vi "AIClient.vi"() -> ()   [LabVIEW 2025]
uses:
  AIGlobalqueue.vi
panel:
  in  "get_action":bool
  out "ACTION":T1
  in  "reset":bool
  out "Numeric 2":i32
  in  "stop":bool
  in  "updateforward":bool
  out "action name":string
  in  "action":i32
  in  "map_size":i32
  out "reset_agent output":i32
  out "action":i32
  out "y":i32
  out "x":i32
  in  "Array 2":i32[](array[numeric])
  out "Array":i32[](array[numeric])
  in  "player_ID":i32
  in  "armies_map":i32[][](array[numeric])
  in  "owner_map":i32[][](array[numeric])
  out "initialize output":i32
  out "error out":errorcluster
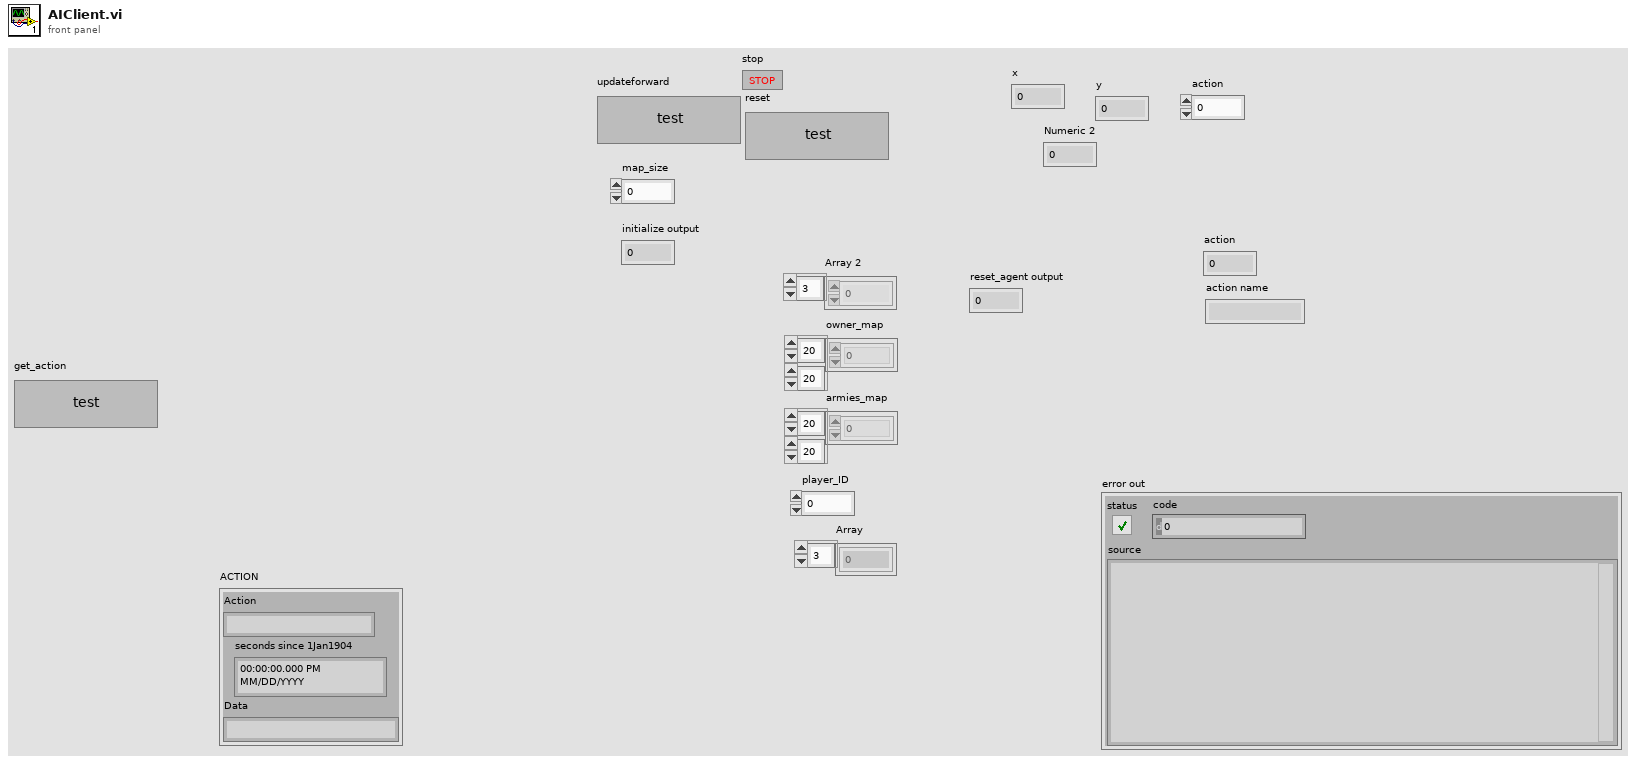
[diagram p1: front panel]
types:
  T1 = cluster{"Action":string, "seconds since 1Jan1904":timestamp, "Data":string}
  T2 = cluster{"seconds since 1Jan1904":timestamp, "Data":string}
  T3 = cluster{"owner_map":i32[][], "armies_map":i32[][], "turn_ID":i32, "player_ID":i32}
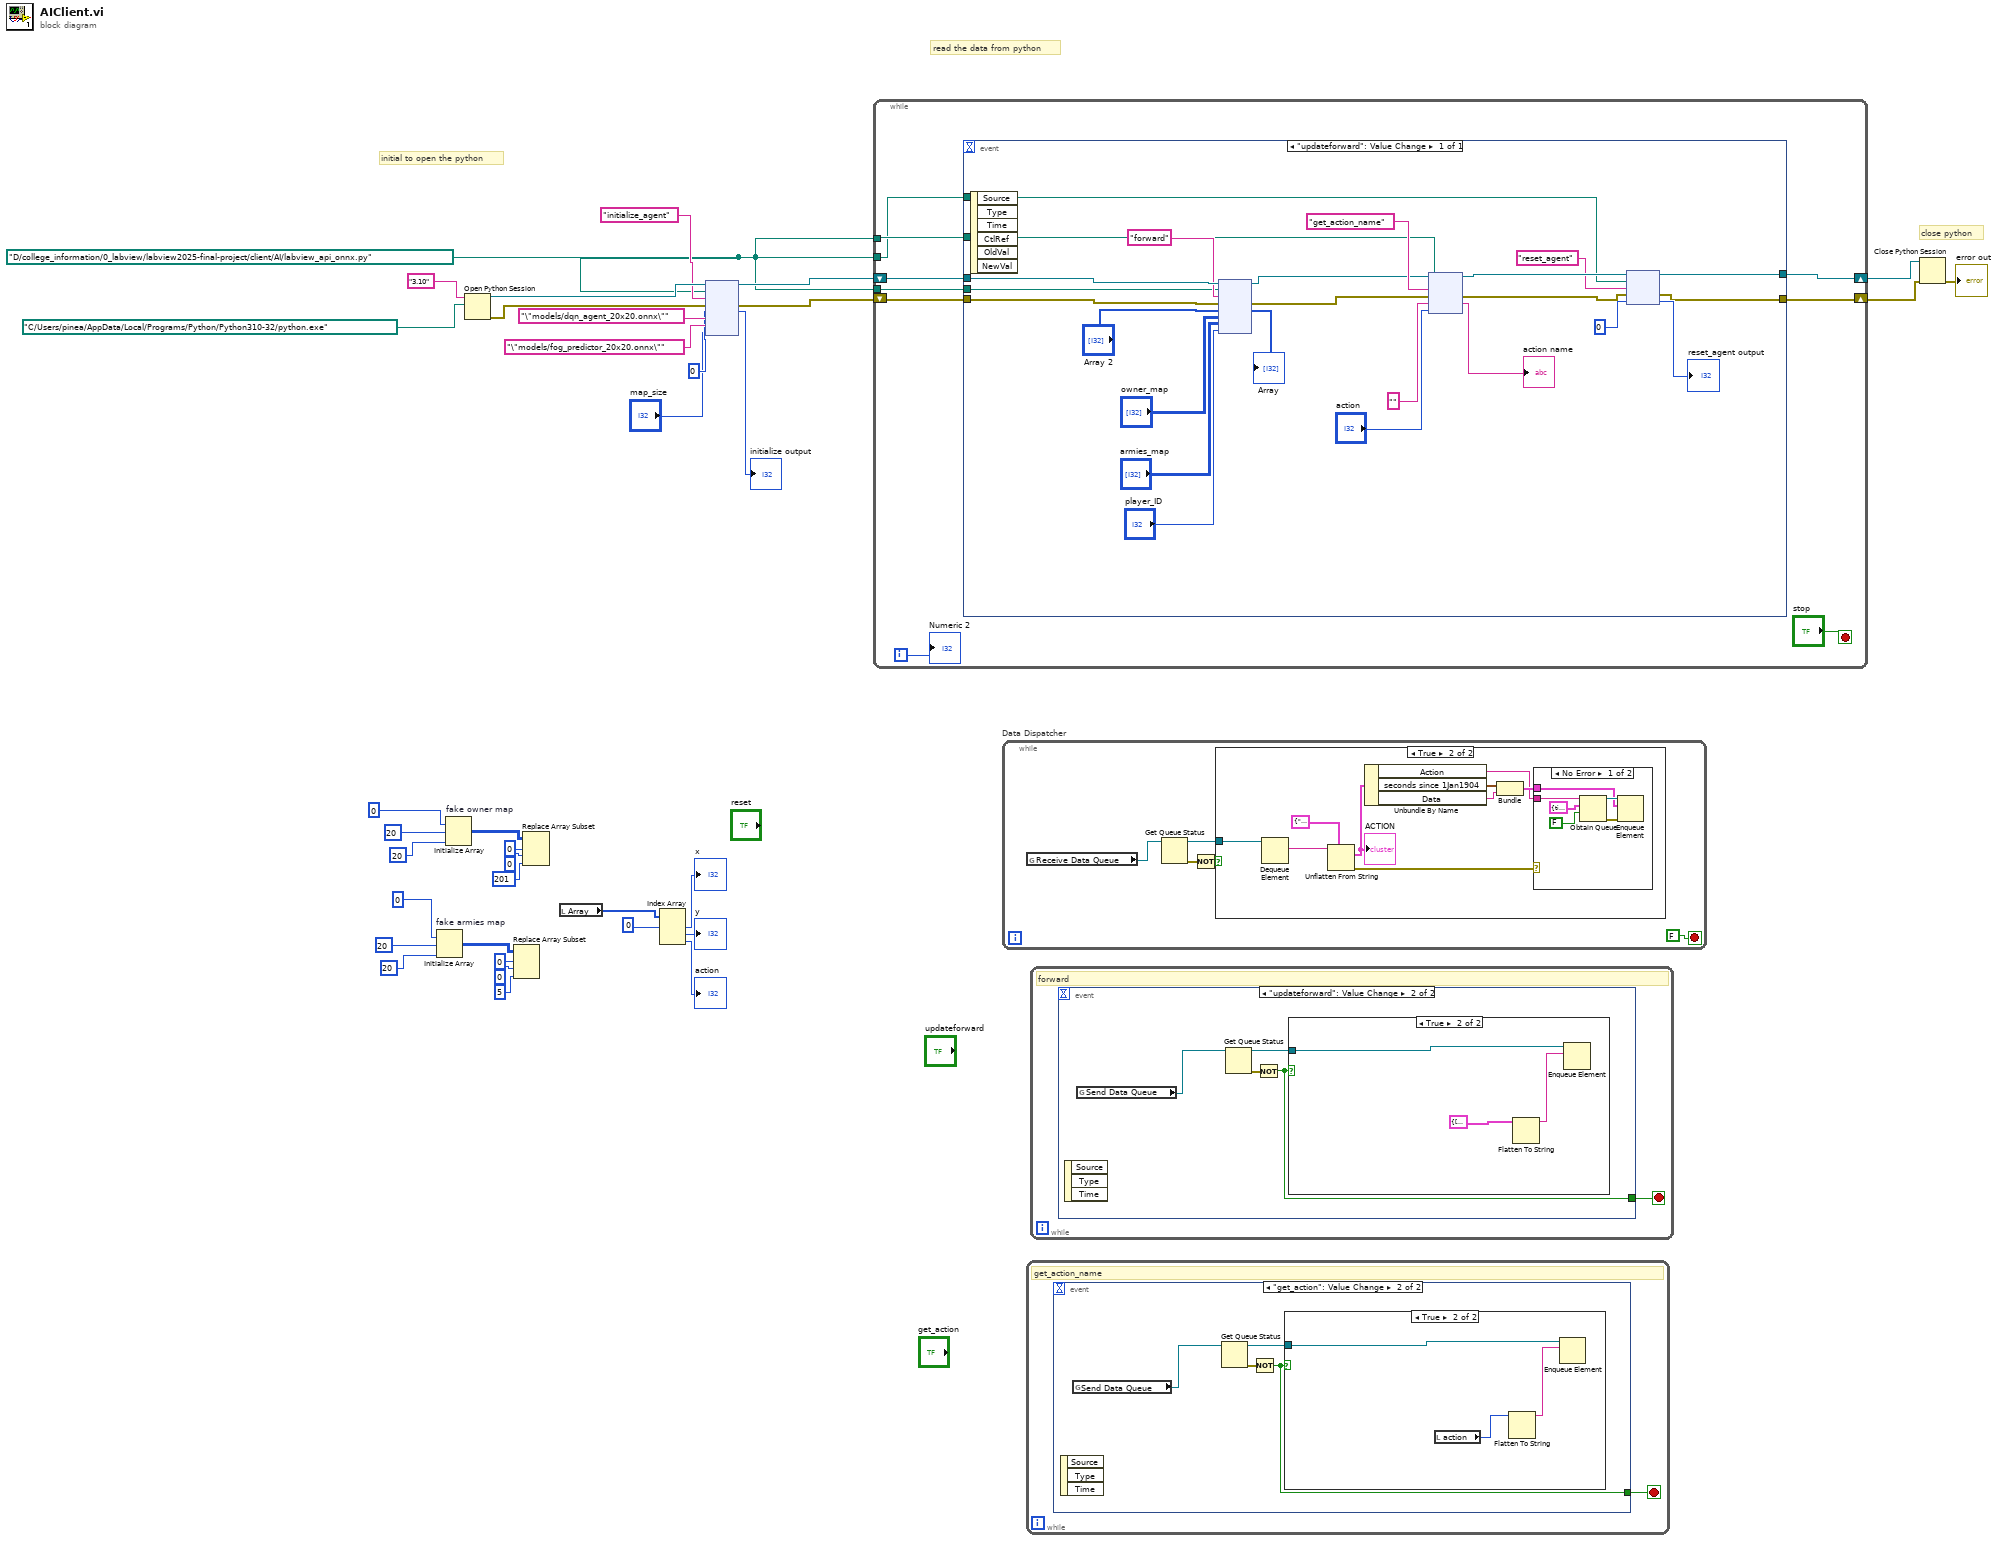
[diagram p0: block diagram]
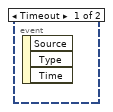
[diagram p2: hidden frame]
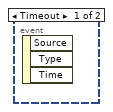
[diagram p4: hidden frame]
diagram:
  w17 = path "D:/college_information/0_labview/labview2025-final-project/client/AI/labview_api_onnx.py" ("Python path")
  # "read the data from python"
  # "close python"
  # "initial to open the python"
  n1 = Initialize Array "fake armies map"(0 ("element"), 20 ("dimension size"), 20 ("dimension size")) -> (w14:i32[][])
  n2 = Initialize Array "fake owner map"(0 ("element"), 20 ("dimension size"), 20 ("dimension size")) -> (w13:i32[][])
  n3 = Open Python Session(python version="3.10" ("Python version"), python path=path "C:/Users/pinea/AppData/Local/Programs/Python/Python310-32/python.exe" ("Python path")) -> (session out=w34:refnum<k35>, error out=w33:errorcluster)  [unwired: 1 in]
  n4 = Replace Array Subset(array=w14, new element=5 ("new element/subarray"), index (row)=0, index (col)=0 ("disabled index (col)")) -> ()  [unwired: 1 out]
  n5 = Replace Array Subset(array=w13, new element=201 ("new element/subarray"), index (row)=0, index (col)=0 ("disabled index (col)")) -> ()  [unwired: 1 out]
  n6 = local read "Array"() -> (w30:i32[])
  n7 = Index Array(array=w30, index #1=0 ("index")) -> (element #1=→"x":i32, element #2=→"y":i32, element #3=→"action":i32)  [unwired: 2 in]
  n8 = node(w34, w17, "initialize_agent" ("function name"), w33, 0, "\"models/dqn_agent_20x20.onnx\"", "\"models/fog_predictor_20x20.onnx\"", "map_size") -> (w20:refnum<k35>, w19:errorcluster, →"initialize output":i32)  [unwired: 3 in, 2 out]
  n9 = while {
    tunnel: w17 -> [w42]
    shift-right: [w37] -> w16
    shift-left: w20 -> [w44]
    shift-right: [w36] -> w15
    shift-left: w19 -> [w43]
    tunnel: w17 -> [w41]
    tunnel: w17 -> [w38]
    i -> [w39]
    stop <- "stop" stop-if-true
    n10 = event shown="[0] \"updateforward\": Value Change" {
      selector: _ -> [_]
      dyn-events: _ -> [_]
      timeout: _ -> [_]
      tunnel: w44 -> [w64]
      tunnel: w43 -> [w63]
      tunnel: w42 -> [w57]
      tunnel: w41 -> [w56]
      tunnel: w38 -> [w53]
      tunnel: [w49] -> w37
      tunnel: [w48] -> w36
      event "updateforward": Value Change {
        n11 = event-data() -> ()  [unwired: 1 in, 6 out]
        n12 = node(w64, w57, "forward" ("function name"), w63, "Array 2", "owner_map", "armies_map", "player_ID") -> (w59:refnum<k35>, w58:errorcluster, →"Array":i32[])  [unwired: 3 in, 2 out]
        n13 = node(w59, w56, "get_action_name" ("function name"), w58, "", "action") -> (w54:refnum<k35>, w51:errorcluster, →"action name":string)  [unwired: 1 in, 2 out]
        n14 = node(w54, w53, "reset_agent" ("function name"), w51, 0) -> (w49:refnum<k35>, w48:errorcluster, →"reset_agent output":i32)  [unwired: 2 out]
      }
    }
    "Numeric 2" <- w39
  }
  n15 = while "Data Dispatcher" {
    stop <- FALSE stop-if-true
    n16 = global read "AIGlobalqueue.vi" "Receive Data Queue"() -> (w69:refnum<queue>)
    n17 = Get Queue Status(queue=w69) -> (queue out=w70:refnum<queue>, error out=w72:errorcluster)  [unwired: 2 in, 6 out]
    n18 = Not(x=w72) -> (.not. x?=w71:bool)
    n19 = case shown="True" w71 {
      tunnel: w70 -> [_ w82]
      frame False {
      }
      frame True {
        n20 = Dequeue Element(queue=w82) -> (element=w81:string)  [unwired: 2 in, 3 out]
        n21 = Unflatten From String(type=T1 {"Action"="", "seconds since 1Jan1904"=timestamp(0 s since 1904-01-01), "Data"=""} ("CommandCluster"), binary string=w81) -> (value=w74:T1, error out=w75:errorcluster)  [unwired: 3 in, 1 out]
        "ACTION" <- w74
        n22 = Unbundle By Name(w74) -> ("Action"=w76:string, "seconds since 1Jan1904"=w79:timestamp, "Data"=w78:string)
        n23 = Bundle("seconds since 1Jan1904"=w79, "Data"=w78) -> (w77:T2)  [unwired: 1 in]
        n24 = case shown="No Error" w75 {
          tunnel: w77 -> [w85 _]
          tunnel: w76 -> [w84 _]
          frame No Error {
            n25 = Obtain Queue(name (unnamed)=w84, element data type=T2 {"seconds since 1Jan1904"=timestamp(0 s since 1904-01-01), "Data"=""} ("ActionDataCluster"), create if not found? (T)=FALSE) -> (queue out=w87:refnum<queue>, error out=w86:errorcluster)  [unwired: 2 in, 1 out]
            n26 = Enqueue Element(queue=w87, element=w85, error in (no error)=w86) -> ()  [unwired: 1 in, 3 out]
          }
          frame Error {
          }
        }
      }
    }
  }
  n27 = while {
    stop <- w89 stop-if-true
    # "get_action_name"
    n28 = event shown="[1] \"get_action\": Value Change" {
      selector: _ -> [_ _]
      dyn-events: _ -> [_ _]
      timeout: _ -> [_ _]
      tunnel: [_ w91] -> w89
      event Timeout {
        n29 = event-data() -> ()  [unwired: 1 in, 3 out]
      }
      event "get_action": Value Change {
        n30 = event-data() -> ()  [unwired: 1 in, 3 out]
        n31 = global read "AIGlobalqueue.vi" "Send Data Queue"() -> (w90:refnum<queue>)
        n32 = Get Queue Status(queue=w90) -> (queue out=w92:refnum<queue>, error out=w93:errorcluster)  [unwired: 2 in, 6 out]
        n33 = Not(x=w93) -> (.not. x?=w91:bool)
        n34 = case shown="True" w91 {
          tunnel: w92 -> [_ w96]
          frame False {
          }
          frame True {
            n35 = local read "action"() -> (w94:i32)
            n36 = Flatten To String(anything=w94) -> (data string=w95:string)  [unwired: 3 in, 2 out]
            n37 = Enqueue Element(queue=w96, element=w95) -> ()  [unwired: 2 in, 3 out]
          }
        }
      }
    }
  }
  n38 = while {
    stop <- w97 stop-if-true
    # "forward"
    n39 = event shown="[1] \"updateforward\": Value Change" {
      selector: _ -> [_ _]
      dyn-events: _ -> [_ _]
      timeout: _ -> [_ _]
      tunnel: [_ w99] -> w97
      event Timeout {
        n40 = event-data() -> ()  [unwired: 1 in, 3 out]
      }
      event "updateforward": Value Change {
        n41 = event-data() -> ()  [unwired: 1 in, 3 out]
        n42 = global read "AIGlobalqueue.vi" "Send Data Queue"() -> (w98:refnum<queue>)
        n43 = Get Queue Status(queue=w98) -> (queue out=w100:refnum<queue>, error out=w101:errorcluster)  [unwired: 2 in, 6 out]
        n44 = Not(x=w101) -> (.not. x?=w99:bool)
        n45 = case shown="True" w99 {
          tunnel: w100 -> [_ w104]
          frame False {
          }
          frame True {
            n46 = Flatten To String(anything=T3 {"owner_map"=[], "armies_map"=[], "turn_ID"=0, "player_ID"=0} ("PlayerInfo")) -> (data string=w103:string)  [unwired: 3 in, 2 out]
            n47 = Enqueue Element(queue=w104, element=w103) -> ()  [unwired: 2 in, 3 out]
          }
        }
      }
    }
  }
  n48 = Close Python Session(session in=w16, error in=w15) -> (11:→"error out":errorcluster)
